vi "DAQ.EnumerateDevices.vi"(8 "error in (no error)":errorcluster) -> (0 "error out":errorcluster, 3 "Devices":T1[](array[typedef]))   [LabVIEW 2019, in "Instrument.Lockin.lvlib" / "Instrument.DAQ.lvclass"]
uses:
  Instrument.DAQ.lvclass
  <resource>/objmgr/daqmx.rc
  Typedefs/DeviceInfo--Cluster.ctl
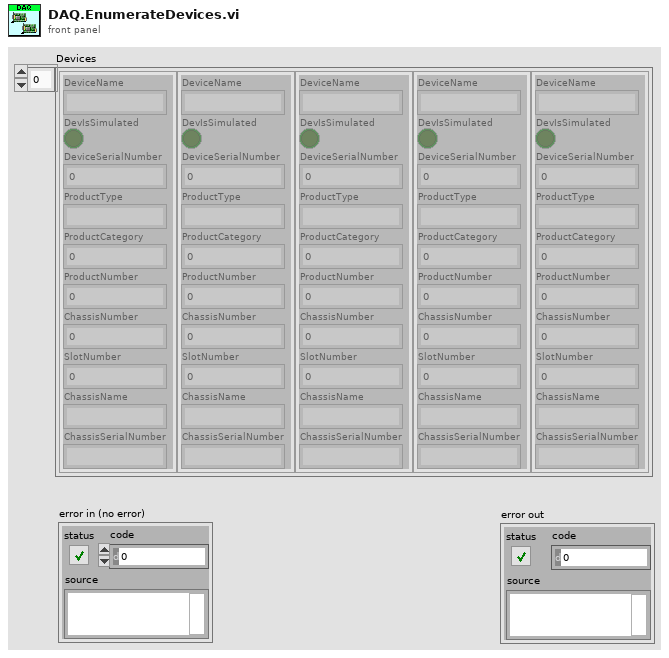
[diagram p1: front panel]
types:
  T1 = typedef "Instrument.Lockin.lvlib/Instrument.DAQ.lvclass/DeviceInfo--Cluster.ctl" = cluster{"DeviceName":string, "DevIsSimulated":bool, "DeviceSerialNumber":u32, "ProductType":string, "ProductCategory":i32, "ProductNumber":u32, "ChassisNumber":u32, "SlotNumber":u32, "ChassisName":string, "ChassisSerialNumber":string}
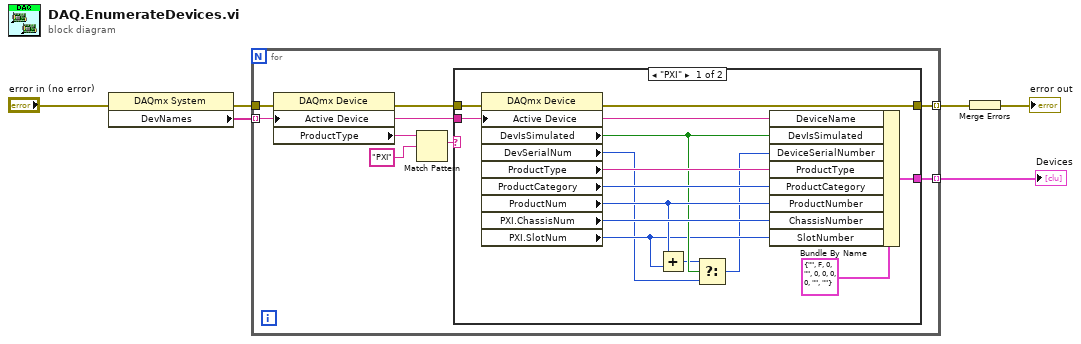
[diagram p0: block diagram]
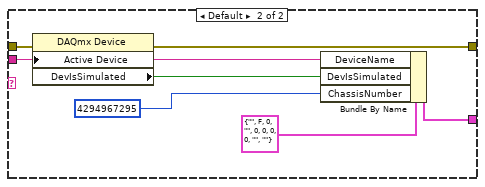
[diagram p2: hidden frame]
diagram:
  n1 = property class="DAQmx System"(error in="error in (no error)") -> (error out=w2:errorcluster, "DevNames"=w3:tag[])  [unwired: 1 in, 1 out]
  n2 = for {
    tunnel: w3 -> [w8] mode=indexing
    tunnel: w2 -> [w14]
    tunnel: [w9] -> w4 mode=indexing
    tunnel: [w7] -> w6 mode=indexing
    n3 = property class="DAQmx Device"(error in=w14, "Active Device"=w8) -> (error out=w10:errorcluster, "ProductType"=w13:string)  [unwired: 1 in, 1 out]
    n4 = Match Pattern(string=w13, regular expression="PXI") -> (match substring=w12:string)  [unwired: 1 in, 3 out]
    n5 = case shown="\"PXI\"" w12 {
      tunnel: w10 -> [w28 w34]
      tunnel: [w27 w35] -> w9
      tunnel: w8 -> [w26 w32]
      tunnel: [w25 w29] -> w7
      frame "PXI" {
        n6 = property class="DAQmx Device"(error in=w28, "Active Device"=w26) -> (error out=w27:errorcluster, "DevIsSimulated"=w19:bool, "DevSerialNum"=w16:u32, "ProductType"=w21:string, "ProductCategory"=w22:i32, "ProductNum"=w20:u32, "PXI.ChassisNum"=w23:u32, "PXI.SlotNum"=w17:u32)  [unwired: 1 in, 1 out]
        n7 = Add(x=w20, y=w17) -> (x+y=w18:u32)
        n8 = Select(t=w18, s=w19, f=w16) -> (s? t:f=w15:u32)
        n9 = Bundle By Name(cluster=T1 {"DeviceName"="", "DevIsSimulated"=FALSE, "DeviceSerialNumber"=0, "ProductType"="", "ProductCategory"=0, "ProductNumber"=0, "ChassisNumber"=0, "SlotNumber"=0, "ChassisName"="", "ChassisSerialNumber"=""} ("Device"), "DeviceName"=w26, "DevIsSimulated"=w19, "DeviceSerialNumber"=w15, "ProductType"=w21, "ProductCategory"=w22, "ProductNumber"=w20, "ChassisNumber"=w23, "SlotNumber"=w17) -> (w25:T1)
      }
      frame Default {
        n10 = property class="DAQmx Device"(error in=w34, "Active Device"=w32) -> (error out=w35:errorcluster, "DevIsSimulated"=w31:bool)  [unwired: 1 in, 1 out]
        n11 = Bundle By Name(cluster=T1 {"DeviceName"="", "DevIsSimulated"=FALSE, "DeviceSerialNumber"=0, "ProductType"="", "ProductCategory"=0, "ProductNumber"=0, "ChassisNumber"=0, "SlotNumber"=0, "ChassisName"="", "ChassisSerialNumber"=""} ("Device"), "DeviceName"=w32, "DevIsSimulated"=w31, "ChassisNumber"=u32 4294967295 ("PXI.ChassisNum")) -> (w29:T1)
      }
    }
  }
  "Devices" <- w6
  n12 = Merge Errors(w4) -> (→"error out":errorcluster)
